vi "Parse Relay Code.vi"(1 "Buffer in":string) -> (0 "relay":string)   [LabVIEW 2019, in "PGC2D.lvlib"]
uses:
  PGC2D.lvlib
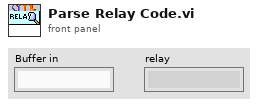
[diagram p1: front panel]
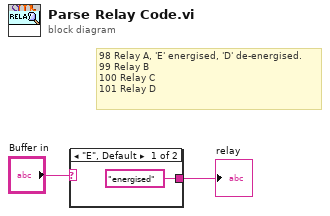
[diagram p0: block diagram]
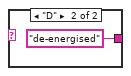
[diagram p2: hidden frame]
diagram:
  # "98 Relay A, 'E' energised, 'D' de-energised.\n99 Relay B\n100 Relay C\n101 Relay D"
  n1 = case shown="\"E\", Default" "Buffer in" {
    tunnel: ["energised" ("replace string (\"\")") "de-energised" ("replace string (\"\")")] -> w2
    frame "E", Default {
    }
    frame "D" {
    }
  }
  "relay" <- w2
